vi "RichToFlatnixnet_grpc_DbMergeResponse.vi"(5 "OutputClusterType":T1, 11 "InputCluster":T2) -> (3 "OutputCluster":T1)   [LabVIEW 2025, in "xnet-grpc_client.lvlib"]
uses:
  nixnet_grpc_DbMergeResponse.ctl
  nixnet_grpc_DbMergeResponse_Flat.ctl
  xnet-grpc_client.lvlib
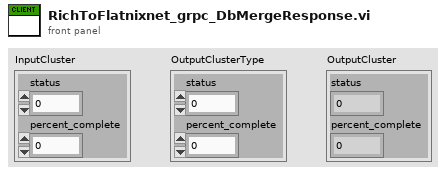
[diagram p1: front panel]
types:
  T1 = typedef "xnet-grpc_client.lvlib/nixnet_grpc_DbMergeResponse_Flat.ctl" = cluster{"status":i32, "percent_complete":u32}
  T2 = typedef "xnet-grpc_client.lvlib/nixnet_grpc_DbMergeResponse.ctl" = cluster{"status":i32, "percent_complete":u32}
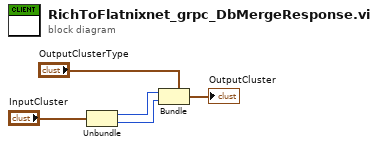
[diagram p0: block diagram]
diagram:
  n1 = Unbundle "Unbundle"("InputCluster") -> ("status"=w2:i32, "percent_complete"=w1:u32)
  n2 = Bundle "Bundle"(cluster="OutputClusterType", "status"=w2, "percent_complete"=w1) -> (→"OutputCluster":T1)
